vi "Get Message.vi"(8 "error in (no error)":errorcluster caption="entrée d'erreur (pas d'erreur)", 10 "Message type":T1="Control", 11 "VIS-IR en entrée":refnum<class "VIS-IR.lvclass">) -> (0 "error out":errorcluster caption="sortie d'erreur", 2 "Message.lvclass":refnum<class "Message.lvclass">, 3 "VIS-IR en sortie":refnum<class "VIS-IR.lvclass">)   [LabVIEW 2015, in "VIS-IR.lvclass"]
uses:
  VIS-IR.lvclass
  Message/Message.lvclass
  dependecies/ControlsVIs/Clusters-def/Message types.ctl
  Detector.lvclass
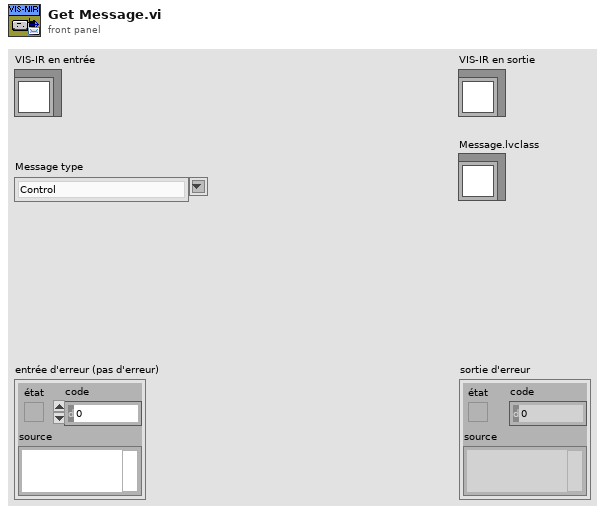
[diagram p1: front panel]
types:
  T1 = typedef "Message types.ctl" = string
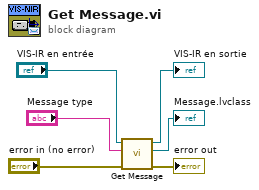
[diagram p0: block diagram]
diagram:
  n1 = call-parent "Get Message.vi"("error in (no error)"="error in (no error)", "Message type"="Message type", "GeneralFunctionality en entrée"="VIS-IR en entrée") -> ("error out"=→"error out":errorcluster, "Message.lvclass"=→"Message.lvclass":refnum<class "Message.lvclass">, "GeneralFunctionality en sortie"=→"VIS-IR en sortie":refnum<class "VIS-IR.lvclass">)  [unwired: 6 in]
